vi "FG Unit Test.vi"() -> ()   [LabVIEW 2018]
uses:
  Custom Controls/Channel.ctl
  Custom Controls/Channel Settings.ctl
  Custom Controls/Waveform Type.ctl
  Function Generator.lvclass/Function Generator.ctl
  Function Generator.lvclass
  Function Generator.lvlib
panel:
  in  "Channel Settings":T1
  in  "Channel":T3
  out "error out":errorcluster
  in  "Stop":bool
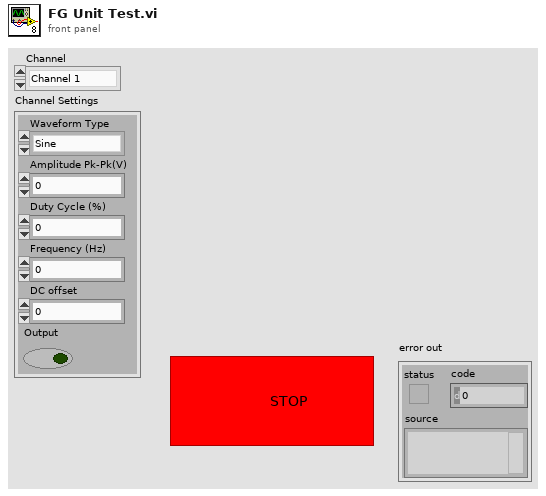
[diagram p1: front panel]
types:
  T1 = typedef "Function Generator.lvlib/Channel Settings.ctl" = cluster{"Waveform Type":T2, "Amplitude Pk-Pk(V)":dbl, "Duty Cycle (%)":dbl, "Frequency (Hz)":dbl, "DC offset":dbl, "Output":bool}
  T2 = typedef "Function Generator.lvlib/Waveform Type.ctl" = enum16{"Sine", "Square", "Triangle", "Sawtooth", "DC"}
  T3 = typedef "Function Generator.lvlib/Channel.ctl" = enum16{"Channel 1", "Channel 2", "Channel 3", "Channel 4"}
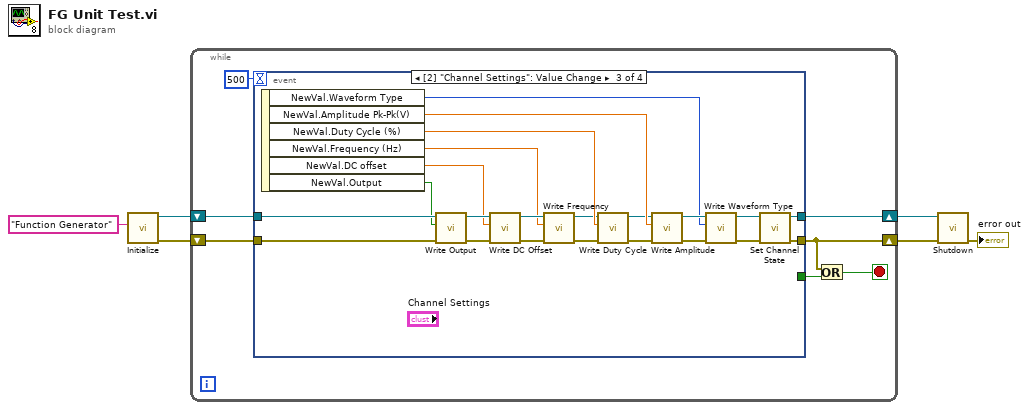
[diagram p0: block diagram]
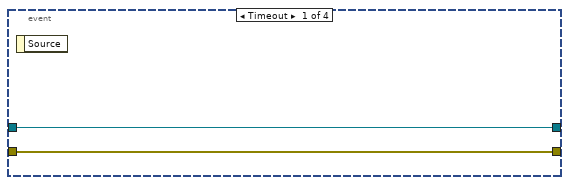
[diagram p2: hidden frame]
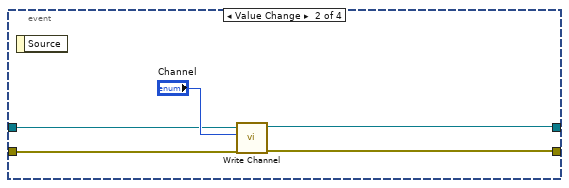
[diagram p3: hidden frame]
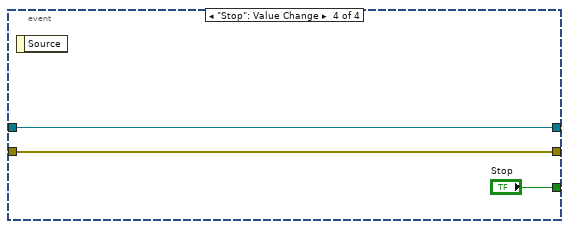
[diagram p4: hidden frame]
diagram:
  n1 = call "Initialize.vi"("Device"="Function Generator") -> ("error out"=w4:errorcluster, "Function Generator out"=w5:refnum<class "Function Generator.lvclass">)  [unwired: 9 in]
  n2 = while {
    shift-right: [w10] -> w2
    shift-left: w5 -> [w13]
    shift-right: [w9] -> w3
    shift-left: w4 -> [w12]
    stop <- w8 stop-if-true
    n3 = event shown="[2] \"Channel Settings\": Value Change" {
      selector: _ -> [_ _ _ _]
      dyn-events: _ -> [_ _ _ _]
      timeout: 500 -> [_ _ _ _]
      tunnel: w13 -> [w15 w19 w29 w44]
      tunnel: w12 -> [w14 w18 w28 w45]
      tunnel: [w15 w17 w41 w44] -> w10
      tunnel: [w14 w16 w42 w45] -> w9
      tunnel: [_ _ _ "Stop"] -> w7
      event Timeout {
        n4 = event-data() -> ()  [unwired: 1 in, 1 out]
      }
      event Value Change {
        n5 = event-data() -> ()  [unwired: 1 in, 1 out]
        n6 = call "Write Channel.vi"("error in (no error)"=w18, "Channel"="Channel", "Function Generator in"=w19) -> ("error out"=w16:errorcluster, "Function Generator out"=w17:refnum<class "Function Generator.lvclass">)  [unwired: 7 in]
      }
      event Value Change {
        n7 = event-data() -> ("NewVal.Waveform Type"=w36:T2, "NewVal.Amplitude Pk-Pk(V)"=w35:dbl, "NewVal.Duty Cycle (%)"=w34:dbl, "NewVal.Frequency (Hz)"=w23:dbl, "NewVal.DC offset"=w22:dbl, "NewVal.Output"=w21:bool)  [unwired: 1 in]
        n8 = call "Write Output.vi"("error in"=w28, "Output"=w21, "Function Generator in"=w29) -> ("error out"=w27:errorcluster, "Function Generator out"=w30:refnum<class "Function Generator.lvclass">)  [unwired: 7 in]
        n9 = call "Write DC Offset.vi"("error in"=w27, "DC Offset"=w22, "Function Generator in"=w30) -> ("error out"=w26:errorcluster, "Function Generator out"=w31:refnum<class "Function Generator.lvclass">)  [unwired: 7 in]
        n10 = call "Write Frequency.vi"("error in"=w26, "Frequency (Hz)"=w23, "Function Generator in"=w31) -> ("error out"=w25:errorcluster, "Function Generator out"=w33:refnum<class "Function Generator.lvclass">)  [unwired: 7 in]
        n11 = call "Write Duty Cycle.vi"("error in"=w25, "Duty Cycle (%)"=w34, "Function Generator in"=w33) -> ("error out"=w24:errorcluster, "Function Generator out"=w32:refnum<class "Function Generator.lvclass">)  [unwired: 7 in]
        n12 = call "Write Amplitude.vi"("error in"=w24, "Amplitude Pk-Pk(V)"=w35, "Function Generator in"=w32) -> ("error out"=w38:errorcluster, "Function Generator out"=w37:refnum<class "Function Generator.lvclass">)  [unwired: 7 in]
        n13 = call "Write Waveform Type.vi"("error in"=w38, "Waveform Type"=w36, "Function Generator in"=w37) -> ("error out"=w39:errorcluster, "Function Generator out"=w40:refnum<class "Function Generator.lvclass">)  [unwired: 7 in]
        n14 = call-dynamic "Set Channel State.vi"("error in (no error)"=w39, "Function Generator in"=w40) -> ("error out"=w42:errorcluster, "Function Generator out"=w41:refnum<class "Function Generator.lvclass">)  [unwired: 8 in]
      }
      event "Stop": Value Change {
        n15 = event-data() -> ()  [unwired: 1 in, 1 out]
      }
    }
    n16 = Or(x=w9, y=w7) -> (x .or. y?=w8:bool)
  }
  n17 = call "Shutdown.vi"("error in"=w3, "Function Generator in"=w2) -> ("error out"=→"error out":errorcluster)  [unwired: 8 in, 1 out]
